vi "Compile Data Refs.vi"(8 "error in":errorcluster, 10 "Execution Unit Information":T5 {"Outgoing Channels" format="%.0x"; "Incoming Channels" format="%.0x"}, 11 "Device Ref in":T4=18446744073709551615 format="%.0x") -> (0 "error out":errorcluster, 2 "Execution Unit Compiled Information":T1 {"Outgoing Data References"."Data Reference" format="%.0x"; "Incoming Data References" format="%.0x"}, 3 "Device Ref out":T4=18446744073709551615 format="%.0x")   [LabVIEW 2020, in "Communication Bus Template System Explorer.lvlib"]
uses:
  Communication Bus Template System Explorer.lvlib
  Includes/Communication Bus Interfaces.lvlibp/Execution Unit/Execution Unit Information.ctl
  Includes/Communication Bus Interfaces.lvlibp/1abvi3w/vi.lib/NI VeriStand/Custom Device API/Custom Device Item Ref.ctl
  <vilib>/NI VeriStand/Custom Device API/Custom Device Item Ref.ctl
  <vilib>/NI VeriStand/Custom Device API/Data Reference.ctl
  <vilib>/NI VeriStand/Custom Device API/Block Data Reference.ctl
  <vilib>/NI VeriStand/Custom Device API/Data Access Type.ctl
  <vilib>/NI VeriStand/Custom Device API/Custom Device API.lvlib
  Shared/Execution Unit Compiled Information.ctl
  Shared/Communication Bus Template Shared.lvlib
  Includes/Communication Bus Interfaces.lvlibp/Execution Unit/Execution Unit/Execution Unit.lvclass
  Includes/Communication Bus Interfaces.lvlibp/1abvi3w/vi.lib/NI VeriStand/Custom Device API/Custom Device API.lvlib
  Includes/Communication Bus Interfaces.lvlibp/Execution Unit/Execution Unit.lvlib
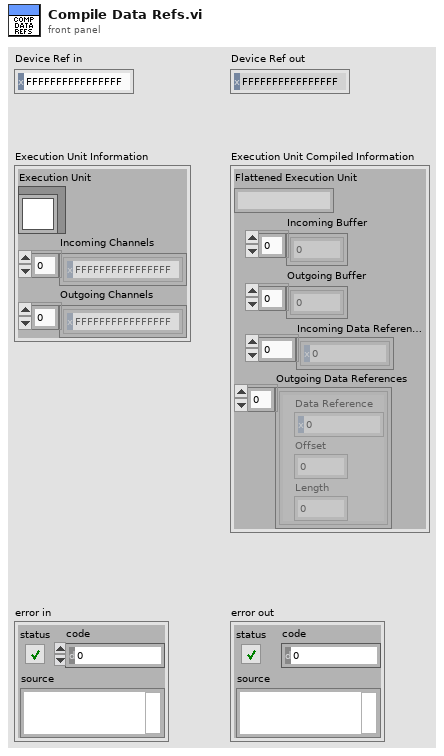
[diagram p1: front panel]
types:
  T1 = typedef "Communication Bus Template Shared.lvlib/Execution Unit Compiled Information.ctl" = cluster{"Flattened Execution Unit":string, "Incoming Buffer":dbl[], "Outgoing Buffer":dbl[], "Incoming Data References":T2[], "Outgoing Data References":T3[]}
  T2 = typedef "Custom Device API.lvlib/Data Reference.ctl" = i32
  T3 = typedef "Custom Device API.lvlib/Block Data Reference.ctl" = cluster{"Data Reference":T2, "Offset":u64, "Length":u64}
  T4 = typedef "Custom Device API.lvlib/Custom Device Item Ref.ctl" = u64
  T5 = typedef "Communication Bus Interfaces.lvlibp/Execution Unit.lvlib/Execution Unit Information.ctl" = cluster{"Execution Unit":refnum<class "Execution Unit.lvclass">, "Incoming Channels":T6[], "Outgoing Channels":T6[]}
  T6 = typedef "Communication Bus Interfaces.lvlibp/Custom Device API.lvlib/Custom Device Item Ref.ctl" = u64
  T7 = typedef "Custom Device API.lvlib/Data Access Type.ctl" = enum16{"Read", "Write"}
  T8 = typedef "Custom Device API.lvlib/Custom Device Channel.ctl" = cluster{"Type":T9, "Units":string, "Default Value":dbl, "Faultable":bool, "Scalable":bool}
  T9 = typedef "Custom Device API.lvlib/Custom Device Channel Type.ctl" = enum16{"Input", "Output"}
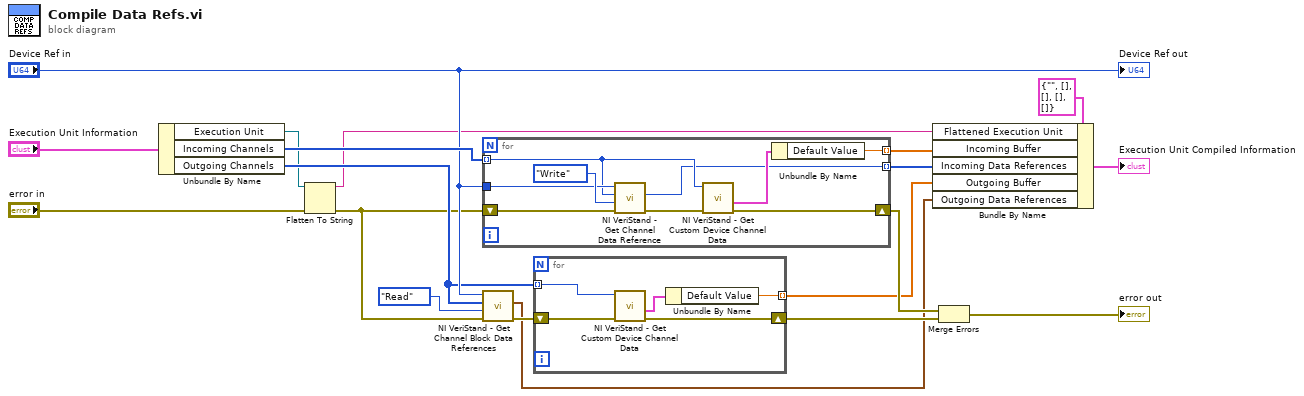
[diagram p0: block diagram]
diagram:
  n1 = Unbundle By Name("Execution Unit Information") -> ("Execution Unit"=w2:refnum<class "Execution Unit.lvclass">, "Incoming Channels"=w19:T6[], "Outgoing Channels"=w14:T6[])
  n2 = Flatten To String(anything=w2, error in (no error)="error in") -> (data string=w1:string, error out=w3:errorcluster)  [unwired: 2 in, 1 out]
  n3 = for {
    tunnel: w19 -> [w25] mode=indexing
    tunnel: "Device Ref in" -> [w27]
    shift-right: [w22] -> w9
    shift-left: w3 -> [w23]
    tunnel: [w21] -> w12 mode=indexing
    tunnel: [w20] -> w11 mode=indexing
    n4 = call <vilib>:"NI VeriStand - Get Channel Data Reference.vi"("error in (no error)"=w23, "Access"=Data_Access_Type."Write", "Channel Ref in"=w25, "Device Ref in"=w27) -> ("error out"=w24:errorcluster, "Channel Data Reference"=w20:T2)  [unwired: 5 in, 1 out]
    n5 = call <vilib>:"NI VeriStand - Get Custom Device Channel Data.vi"("error in (no error)"=w24, "Channel Ref in"=w25) -> ("error out"=w22:errorcluster, "Channel"=w26:T8)  [unwired: 4 in, 4 out]
    n6 = Unbundle By Name(w26) -> ("Default Value"=w21:dbl)
  }
  n7 = call <vilib>:"NI VeriStand - Get Channel Block Data References.vi"("error in (no error)"=w3, "Access"=Data_Access_Type."Read", "Channel Refs"=w14, "Device Ref in"="Device Ref in") -> ("error out"=w15:errorcluster, "Block Data Refs"=w7:T3[])  [unwired: 4 in, 2 out]
  n8 = for {
    shift-right: [w32] -> w8
    shift-left: w15 -> [w33]
    tunnel: w14 -> [w31] mode=indexing
    tunnel: [w29] -> w6 mode=indexing
    n9 = call <vilib>:"NI VeriStand - Get Custom Device Channel Data.vi"("error in (no error)"=w33, "Channel Ref in"=w31) -> ("error out"=w32:errorcluster, "Channel"=w30:T8)  [unwired: 4 in, 4 out]
    n10 = Unbundle By Name(w30) -> ("Default Value"=w29:dbl)
  }
  n11 = Bundle By Name(cluster=T1 {"Flattened Execution Unit"="", "Incoming Buffer"=[], "Outgoing Buffer"=[], "Incoming Data References"=[], "Outgoing Data References"=[]} ("Execution Unit Compiled Information"), "Flattened Execution Unit"=w1, "Incoming Buffer"=w12, "Incoming Data References"=w11, "Outgoing Buffer"=w6, "Outgoing Data References"=w7) -> (→"Execution Unit Compiled Information":T1)
  n12 = Merge Errors(w9, w8) -> (→"error out":errorcluster)
  "Device Ref out" <- "Device Ref in"
